vi "Config Step Sweep.vi"(0 "VISA Resource Name":refnum<visa-resource-name>, 1 "Amplitude Start (-135.00)":dbl=-135.0 format="%.2f", 2 "Amplitude Stop (-135.00)":dbl=-135.0 format="%.2f", 3 "# Points (2)":i32=2, 5 "Frequency Start (1000.00)":dbl=1000.0 format="%.5f", 7 "Frequency Stop (1000.00)":dbl=1000.0 format="%.5f", 9 "Step Dwell (2.00)":dbl=2.0 format="%.2f", 11 "error in (no error)":errorcluster {"code" format="%.0x"}) -> (4 "VISA Resource Name Out":refnum<visa-resource-name>, 15 "error out":errorcluster {"code" format="%.0x"})   [LabVIEW 2014, in "Agilent ESG Series.lvlib"]
doc: "This VI is used to set the controls and the parameters associated with frequency and/or power step sweep."
uses:
  Agilent ESG Series.lvlib
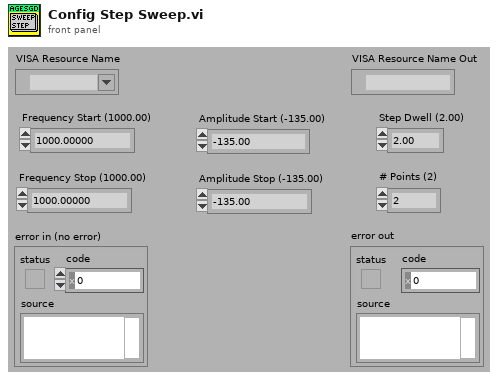
[diagram p1: front panel]
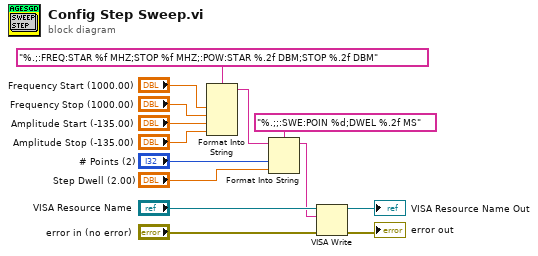
[diagram p0: block diagram]
diagram:
  n1 = Format Into String(format string="%.;:FREQ:STAR %f MHZ;STOP %f MHZ;:POW:STAR %.2f DBM;STOP %.2f DBM", "Frequency Start (1000.00)", "Frequency Stop (1000.00)", "Amplitude Start (-135.00)", "Amplitude Stop (-135.00)") -> (resulting string=w4:string)  [unwired: 2 in, 1 out]
  n2 = Format Into String(format string="%.;;:SWE:POIN %d;DWEL %.2f MS", initial string=w4, "# Points (2)", "Step Dwell (2.00)") -> (resulting string=w1:string)  [unwired: 1 in, 1 out]
  n3 = VISA Write(VISA resource name="VISA Resource Name", write buffer=w1, error in (no error)="error in (no error)") -> (VISA resource name out=→"VISA Resource Name Out":refnum<visa-resource-name>, error out=→"error out":errorcluster)  [unwired: 1 out]
